vi "Get Source and Configuration Channels.vi"(11 "All Endpoint Configurations":T1[](array[typedef])) -> (2 "Configuration Channels":string[](array[string]), 3 "Source Channels":string[](array[string]))   [LabVIEW 2020, in "NI-SWITCH System Explorer.lvlib"]
uses:
  NI-SWITCH System Explorer.lvlib
  Shared/Endpoint Configuration Cluster.ctl
  Shared/Endpoint Configuration Enum.ctl
  Shared/NI-SWITCH Shared.lvlib
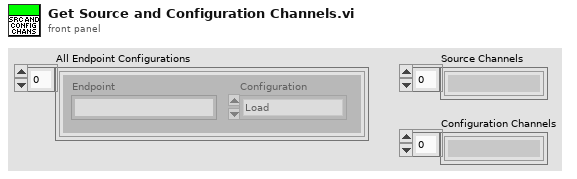
[diagram p1: front panel]
types:
  T1 = typedef "NI-SWITCH Shared.lvlib/Endpoint Configuration Cluster.ctl" = cluster{"Endpoint":string, "Configuration":T2}
  T2 = typedef "NI-SWITCH Shared.lvlib/Endpoint Configuration Enum.ctl" = enum16{"Load", "Source", "Configuration"}
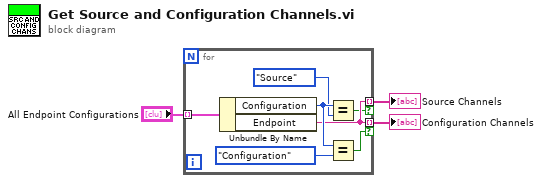
[diagram p0: block diagram]
diagram:
  n1 = for {
    tunnel: "All Endpoint Configurations" -> [w10] mode=indexing
    tunnel: [w8] -> w3 mode=indexing if=w6
    tunnel: [w8] -> w2 mode=indexing if=w7
    n2 = Unbundle By Name(w10) -> ("Configuration"=w9:T2, "Endpoint"=w8:string)
    n3 = Equal?(x=w9, y=Endpoint_Configuration_Enum."Source") -> (x = y?=w7:bool)
    n4 = Equal?(x=w9, y=Endpoint_Configuration_Enum."Configuration") -> (x = y?=w6:bool)
  }
  "Configuration Channels" <- w3
  "Source Channels" <- w2
